vi "Settings AH2700A (SubVI).vi"(4 "Units":i32(ring)=1 items=["nanosiemens"=1, "dissipation factor"=2, "kilohms"=3, "gigohms"=4, "loss vector (jpF)"=5], 5 "Maximum Voltage":dbl=0.01 min=0.0003 max=15.0 step=1.0 format="%#.6f", 6 "Frequency":dbl(ring)=1000.0 items=["50"=50.0, "60"=60.0, "70"=70.0, "80"=80.0, "100"=100.0, "120"=120.0, "140"=140.0, "160"=160.0, "200"=200.0, "240"=240.0, "300"=300.0, "400"=400.0, "500"=500.0, "600"=600.0, "700"=700.0, "800"=800.0, "1000"=1000.0, "1200"=1200.0, "1400"=1400.0, "1600"=1600.0, "2000"=2000.0, "2400"=2400.0, "3000"=3000.0, "4000"=4000.0, "5000"=5000.0, "6000"=6000.0, "7000"=7000.0, "8000"=8000.0, "10000"=10000.0, "12000"=12000.0, "14000"=14000.0, "16000"=16000.0, "20000"=20000.0], 7 "DC Bias":T2(ring), 8 "error in":errorcluster, 10 "Average Exponent":u16=4 max=15, 11 "Instrument parameters (in)":T1) -> (0 "error out":errorcluster, 3 "Instrument parameters (out)":T1)   [LabVIEW 2025]
uses:
  TYPE DEFS/S2DS_Instrument parameters.ctl
panel:
  in  "Boolean 4":bool
  in  "Boolean 3":bool
  out "error":errorcluster
  in  "Boolean 2":bool
  in  "Boolean":bool
  out "Voltage":dbl
  out "Units":i32(ring) items=["", "nanosiemens", "dissipation factor", "kilohms", "gigohms", "loss vector (jpF)"]
  out "Loss":dbl format="%#_10f"
  out "Capacitance":dbl format="%#_10f"
  out "Frequency":dbl
  # "AH 2700A Capacitance bridge settings"
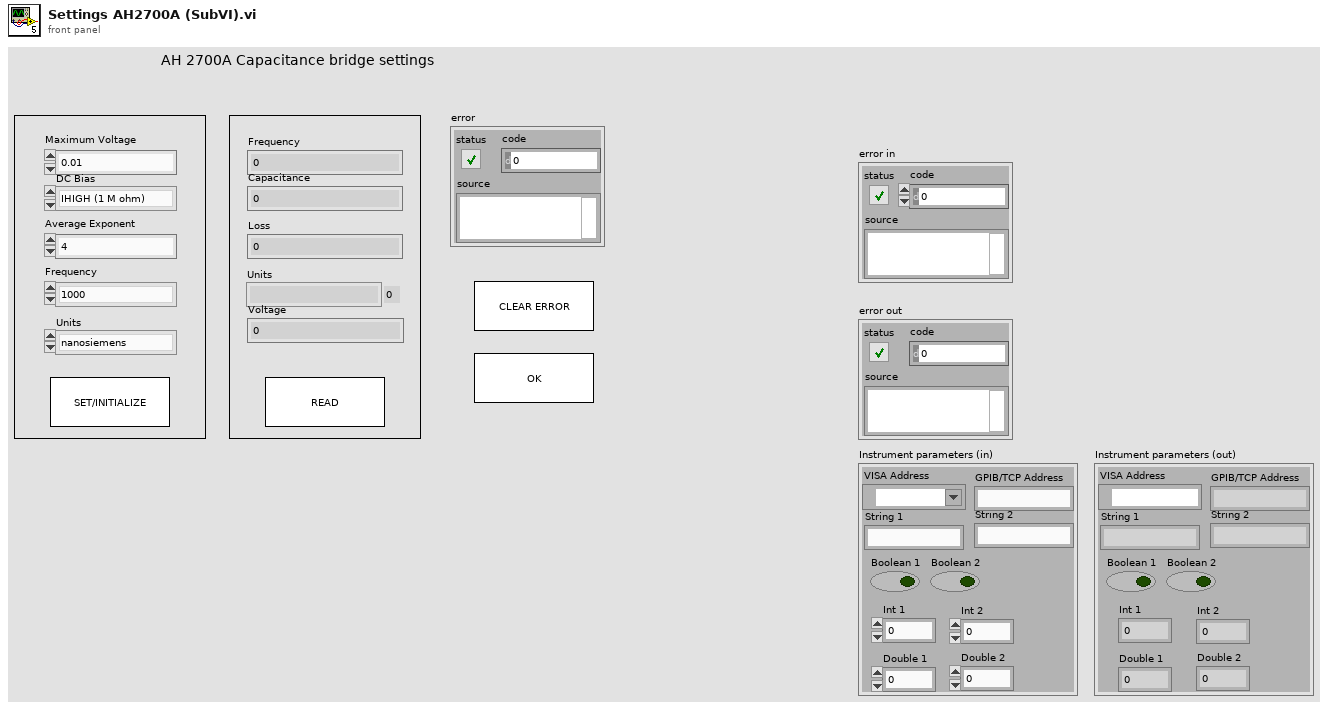
[diagram p1: front panel]
types:
  T1 = typedef "S2DS_Instrument parameters.ctl" = cluster{"VISA Address":refnum<visa-resource-name>, "GPIB/TCP Address":string, "String 1":string, "String 2":string, "Boolean 1":bool, "Boolean 2":bool, "Int 1":i32, "Int 2":i32, "Double 1":dbl, "Double 2":dbl}
  T2 = enum16{"IHIGH (1 M ohm)", "ILOW (100 M ohm)", "OFF"}
  T3 = cluster{"Baud Rate":u32, "Parity":u16, "Data Bits":u16, "Stop Bits":u16}
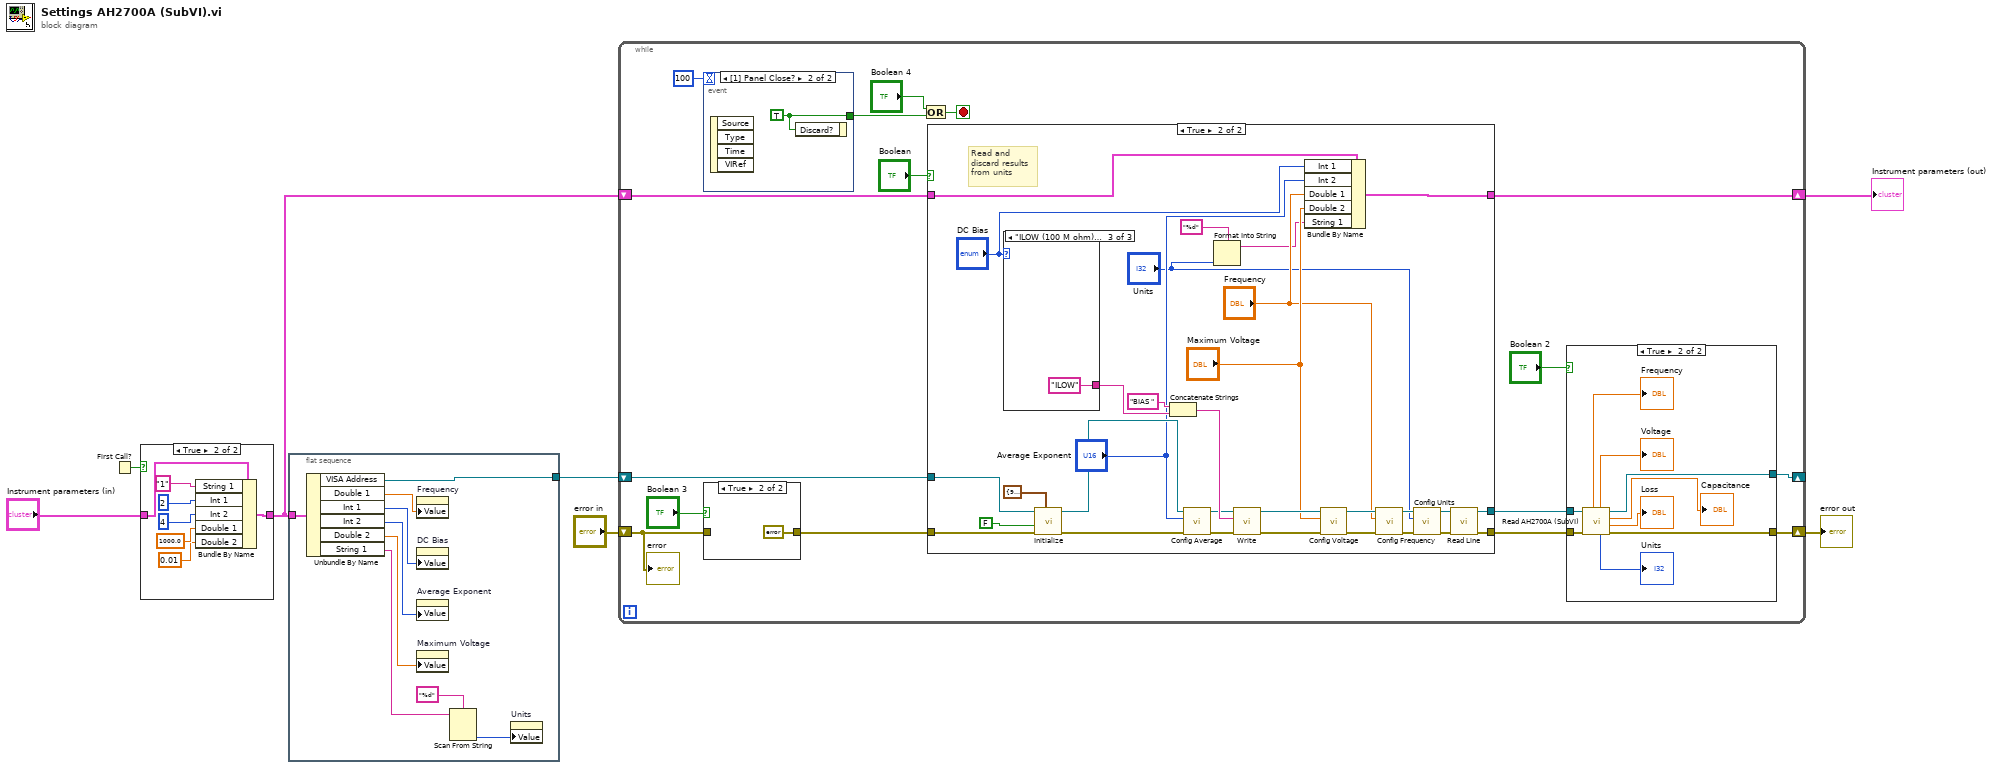
[diagram p0: block diagram]
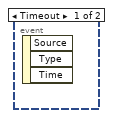
[diagram p5: hidden frame]
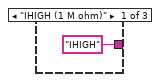
[diagram p7: hidden frame]
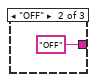
[diagram p8: hidden frame]
diagram:
  n1 = First Call?() -> (First Call?: T/F=w3:bool)
  n2 = case shown="True" w3 {
    tunnel: [w8 w14] -> w1
    tunnel: "Instrument parameters (in)" -> [w8 w15]
    frame False {
    }
    frame True {
      n3 = Bundle By Name(cluster=w15, "String 1"="1", "Int 1"=2, "Int 2"=4, "Double 1"=1000.0, "Double 2"=0.01) -> (w14:T1)
    }
  }
  n4 = flat-sequence {
    tunnel: w1 -> [w24]
    tunnel: [w23] -> w5
    frame #0 {
      n5 = Unbundle By Name(w24) -> ("VISA Address"=w23:refnum<visa-resource-name>, "Double 1"=w22:dbl, "Int 1"=w19:i32, "Int 2"=w21:i32, "Double 2"=w20:dbl, "String 1"=w18:string)
      n6 = property on="Frequency" class="Ring (strict)"("Value"=w22) -> ()  [unwired: 2 in, 2 out]
      n7 = property on="DC Bias" class="Enum (strict)"("Value"=w19) -> ()  [unwired: 2 in, 2 out]
      n8 = property on="Average Exponent" class="DigNum (strict)"("Value"=w21) -> ()  [unwired: 2 in, 2 out]
      n9 = property on="Maximum Voltage" class="DigNum (strict)"("Value"=w20) -> ()  [unwired: 2 in, 2 out]
      n10 = Scan From String(format string="%d", input string=w18) -> (output 1=w16:i32)  [unwired: 3 in, 3 out]
      n11 = property on="Units" class="Ring (strict)"("Value"=w16) -> ()  [unwired: 2 in, 2 out]
    }
  }
  n12 = while {
    shift-right: [w35] -> _
    shift-left: w5 -> [w36]
    shift-right: [w34] -> w7
    shift-left: "error in" -> [w32]
    shift-right: [w26] -> w4
    shift-left: w1 -> [w25]
    stop <- w27 stop-if-true
    n13 = event shown="[1] Panel Close?" {
      selector: _ -> [_ _]
      dyn-events: _ -> [_ _]
      timeout: 100 -> [_ _]
      tunnel: [_ w54] -> w29
      event Timeout {
        n14 = event-data() -> ()  [unwired: 1 in, 3 out]
      }
      event Panel Close? {
        w54 = TRUE ("Discard?")
        n15 = event-data() -> ()  [unwired: 1 in, 4 out]
        n16 = event-data("Discard?"=w54) -> ()  [unwired: 1 in, 1 out]
      }
    }
    n17 = case shown="True" "Boolean 3" {
      tunnel: [w41 errorcluster {"status"=FALSE, "code"=0, "source"=""} ("error in")] -> w31
      tunnel: w32 -> [w41 _]
      frame False {
      }
      frame True {
      }
    }
    n18 = Or(x="Boolean 4", y=w29) -> (x .or. y?=w27:bool)
    n19 = case shown="True" "Boolean" {
      tunnel: [w57 w70] -> w40
      tunnel: [w56 w69] -> w39
      tunnel: w36 -> [w57 w68]
      tunnel: w31 -> [w56 w67]
      tunnel: [w55 w65] -> w26
      tunnel: w25 -> [w55 w66]
      frame False {
      }
      frame True {
        # "Read and\ndiscard results\nfrom units"
        n20 = case shown="\"ILOW (100 M ohm)\", Default" "DC Bias" {
          tunnel: ["IHIGH" "OFF" "ILOW"] -> w86
          frame "IHIGH (1 M ohm)" {
          }
          frame "OFF" {
          }
          frame "ILOW (100 M ohm)", Default {
          }
        }
        n21 = call "Initialize.vi"("Serial Configuration"=T3 {"Baud Rate"=9600, "Parity"=0, "Data Bits"=8, "Stop Bits"=10}, "error in (no error)"=w67, "Reset (True)"=FALSE, "VISA resource name"=w68) -> ("error out"=w79:errorcluster, "VISA resource name out"=w78:refnum<visa-resource-name>)  [unwired: 6 in]
        n22 = Concatenate Strings("BIAS " ("string"), w86) -> (w87:string)
        n23 = call "Config Average.vi"("error in"=w79, "Average Exponent (4)"="Average Exponent", "VISA resource name"=w78) -> ("error out"=w83:errorcluster, "VISA resource name out"=w81:refnum<visa-resource-name>)  [unwired: 7 in]
        n24 = Format Into String(format string="%d", "Units") -> (resulting string=w58:string)  [unwired: 2 in, 1 out]
        n25 = call "Write.vi"("error in"=w83, "command"=w87, "VISA resource name"=w81) -> ("error out"=w84:errorcluster, "VISA resource name out"=w82:refnum<visa-resource-name>)  [unwired: 7 in]
        n26 = Bundle By Name(cluster=w66, "Int 1"="DC Bias", "Int 2"="Average Exponent", "Double 1"="Frequency", "Double 2"="Maximum Voltage", "String 1"=w58) -> (w65:T1)
        n27 = call "Config Voltage.vi"("error in"=w84, "Voltage (15 V)"="Maximum Voltage", "VISA resource name"=w82) -> ("error out"=w74:errorcluster, "VISA resource name out"=w72:refnum<visa-resource-name>)  [unwired: 7 in]
        n28 = call "Config Frequency.vi"("error in"=w74, "Frequency (1000 Hz)"="Frequency", "VISA resource name"=w72) -> ("error out"=w75:errorcluster, "VISA resource name out"=w73:refnum<visa-resource-name>)  [unwired: 7 in]
        n29 = call "Config Units.vi"("error in"=w75, "Units (nS)"="Units", "VISA resource name"=w73) -> ("error out"=w77:errorcluster, "VISA resource name out"=w76:refnum<visa-resource-name>)  [unwired: 7 in]
        n30 = call "Read Line.vi"("error in"=w77, "VISA resource name"=w76) -> ("error out"=w69:errorcluster, "VISA resource name out"=w70:refnum<visa-resource-name>)  [unwired: 5 in, 3 out]
      }
    }
    n31 = case shown="True" "Boolean 2" {
      tunnel: w40 -> [w44 w53]
      tunnel: w39 -> [w43 w52]
      tunnel: [w44 w46] -> w35
      tunnel: [w43 w45] -> w34
      frame False {
      }
      frame True {
        n32 = call "Read AH2700A (SubVI).vi"("error in (no error)"=w52, "VISA Refnum in"=w53) -> ("error out"=w45:errorcluster, "Loss"=→"Loss":dbl, "Capacitance"=→"Capacitance":dbl, "VISA Refnum out"=w46:refnum<visa-resource-name>, "Units 2"=→"Units":i32, "Voltage"=→"Voltage":dbl, "Frequency"=→"Frequency":dbl)  [unwired: 3 in]
      }
    }
    "error" <- w32
  }
  "error out" <- w7
  "Instrument parameters (out)" <- w4
